vi "transmit.vi"(8 "error in (no error)":errorcluster, 11 "ILCCommunications in":refnum<class "ILCCommunications.lvclass">) -> (0 "error out":errorcluster, 3 "ILCCommunications out":refnum<class "ILCCommunications.lvclass">)   [LabVIEW 2016, in "ILCCommunications.lvclass"]
uses:
  ILCCommunications.lvclass
  ILCCommunications.lvclass/ILCCommunications.ctl
  Common_RT_Modbus/IModbus/IModbus.lvclass
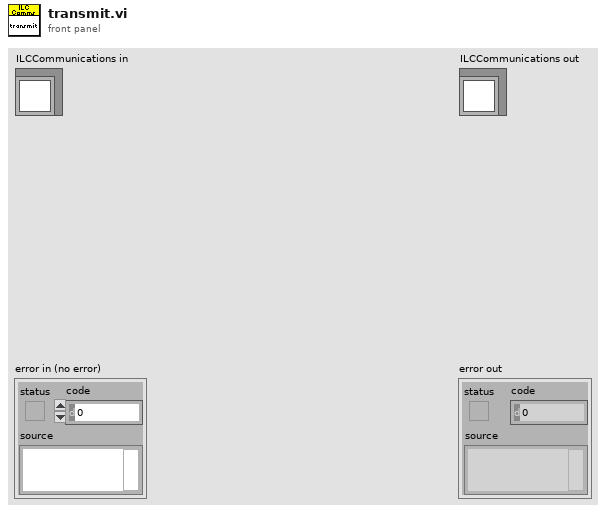
[diagram p1: front panel]
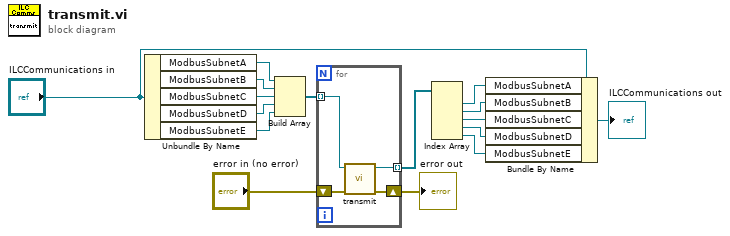
[diagram p0: block diagram]
diagram:
  n1 = Unbundle By Name("ILCCommunications in") -> ("ModbusSubnetA"=w16:refnum<class "IModbus.lvclass">, "ModbusSubnetB"=w15:refnum<class "IModbus.lvclass">, "ModbusSubnetC"=w14:refnum<class "IModbus.lvclass">, "ModbusSubnetD"=w13:refnum<class "IModbus.lvclass">, "ModbusSubnetE"=w12:refnum<class "IModbus.lvclass">)
  n2 = Build Array(w16, w15, w14, w13, w12) -> (w11:refnum<class "IModbus.lvclass">[])
  n3 = for {
    tunnel: w11 -> [w20] mode=indexing
    tunnel: [w19] -> w10 mode=indexing
    shift-right: [w17] -> w1
    shift-left: "error in (no error)" -> [w18]
    n4 = call-dynamic "transmit.vi"("error in (no error)"=w18, "IModbus in"=w20) -> ("error out"=w17:errorcluster, "IModbus out"=w19:refnum<class "IModbus.lvclass">)  [unwired: 8 in]
  }
  "error out" <- w1
  n5 = Index Array(array=w10) -> (element #1=w7:refnum<class "IModbus.lvclass">, element #2=w6:refnum<class "IModbus.lvclass">, element #3=w5:refnum<class "IModbus.lvclass">, element #4=w4:refnum<class "IModbus.lvclass">, element #5=w3:refnum<class "IModbus.lvclass">)  [unwired: 5 in]
  n6 = Bundle By Name(cluster="ILCCommunications in", "ModbusSubnetA"=w7, "ModbusSubnetB"=w6, "ModbusSubnetC"=w5, "ModbusSubnetD"=w4, "ModbusSubnetE"=w3) -> (→"ILCCommunications out":refnum<class "ILCCommunications.lvclass">)
